vi "waveformexample.vi"() -> ()   [LabVIEW 2015]
panel:
  out "Waveform Chart":dynamicdata(graph)
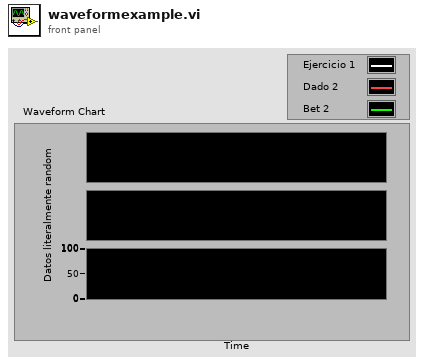
[diagram p1: front panel]
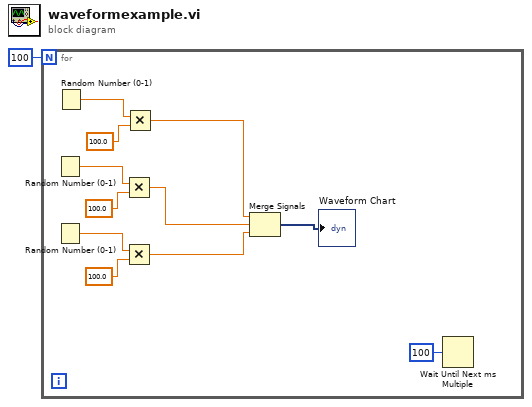
[diagram p0: block diagram]
diagram:
  n1 = for {
    N: 100 -> [_]
    n2 = Random Number (0-1)() -> (number: 0 to 1=w8:dbl)
    n3 = Random Number (0-1)() -> (number: 0 to 1=w5:dbl)
    n4 = Random Number (0-1)() -> (number: 0 to 1=w11:dbl)
    n5 = Multiply(x=w8, y=100.0) -> (x*y=w3:dbl)
    n6 = Multiply(x=w5, y=100.0) -> (x*y=w2:dbl)
    n7 = Multiply(x=w11, y=100.0) -> (x*y=w4:dbl)
    n8 = Merge Signals(w4, w3, w2) -> (→"Waveform Chart":dynamicdata)
    n9 = Wait Until Next ms Multiple(millisecond multiple=u32 100) -> ()  [unwired: 1 out]
  }
